vi "ProstateThumbnails.vi"(5 "Log scaling?":bool, 6 "single frame?":bool, 7 "Data":i16[][][](array[numeric]), 9 "Overlay Co-Ords":T2 {"y overlay" format="%.2f"; "x overlay" format="%.2f"}, 10 "output cluster":T1={"header info"={"Header"="", "Head length"=0}, "A/D info"={"# rf points per line"=0, "# lines per scan"=0, "sample rate MHz"=0, "# A/D bits"=0, "# bytes per A/D"=0, "TGC Flag"=0, "A/D Type"=""}, "Tranducer Info"={"bandwidth"=0.0, "center freq"=0.0, "start freq"=0.0, "ID"=0}, "Scan Info"={"delay"=0.0, "pivot distance"=0.0, "sector scan angle"=0.0, "operator"="", "Scan Mode"="", "location"=""}, "Time/Date Info"={"date"="", "time"=""}, "RF Info"={"RF file name"="", "RF file att"="", "RF cal file name"="", "RF cal file att"=""}, "Patient Info"={"ID"="", "extended ID"="", "age"=0, "sex"="", "previously\nscanned"="", "PSA"=0.0, "LOS"=1, "Ethnicty 2"=3, "Race"=3}, "Tissue Type"={"organ"=0, "disease type"=0, "disease location"=0, "IQ_pts"=0, "RcvBuffer"=0, "RcvFrame"=0, "IQBuff"=0, "IQFrame"=0, "IQPage"=0}, "Votage scaling"={"Digitizer (dB)"=0.0, "Gain (dB)"=0.0, "Atten (dB)"=0.0}, "Comment"="", "Misc Info"={"avg num"=0, "c speed"=0, "Div By or SF zones"=0, "XMIT CHS"=0, "RCV CHS"=0, "Xmit angle"=0.0}, "Therapy Parameters"={"Theraputic Freq (MHz)"=0.1, "Time on (s)"=1.0, "Therapy amplitude (mV)"=50.0, "Lines Before"=20, "Lines After"=80}, "Scan Settings"={"Energy (uJ or V)"=0, "Damp (Ohm) or Fc"=0, "HP Filt (KHz)"=0, "LP Filt (MHz)"=0, "Gain (db)"=0, "prf (kHz)"=0.0, "Distance between\nscan lines (um)"=0, "Distance between\nscan planes (um)"=0, "Scan line gap (um)"=0.0, "Scan plane gap (um)"=0.0}, "Compression Parameters"={"F1 (MHz)"=0.0, "F2 (MHz)"=0.0, "% taper"=0.0, "duration"=0.0}, "Patient Info Xtra"={"First Name"="", "Last Name"="", "Notes"=""}, "ROI Box"=[0, 0, 0, 0]} {"Compression Parameters"."% taper" min=50 max=1000 format="%.2f"; "Compression Parameters"."F2 (MHz)" format="%.3f"; "Compression Parameters"."F1 (MHz)" format="%.3f"; "Scan Settings"."prf (kHz)" format="%.2f"; "Therapy Parameters"."Therapy amplitude (mV)" min=50 max=1000 format="%.2f"; "Therapy Parameters"."Time on (s)" format="%.3f"; "Therapy Parameters"."Theraputic Freq (MHz)" format="%.3f"; "Patient Info"."Race" items=["Am Ind or Alaska", "Asian", "Hawaiian, Pac Isl", "Black or Afr Amer", "White", "more than one race", "unknown"]; "Patient Info"."Ethnicty 2" items=["Hispanic", "Non-Hispanic", "unknown"]; "Patient Info"."LOS" items=["1", "2", "3", "4", "5"]; "Patient Info"."PSA" format="%.1f"; "Scan Info"."delay" format="%.2f"; "Scan Info"."pivot distance" format="%.2f"; "Scan Info"."sector scan angle" format="%.2f"; "Tranducer Info"."bandwidth" format="%.2f"; "Tranducer Info"."center freq" format="%.2f"; "Tranducer Info"."start freq" format="%.2f"}, 11 "Thumb Size":cluster{"pixels in x":i16, "pixels in y":i16}) -> (3 "Thumbs out":picture[](array[picture]))   [LabVIEW 2022 SP3]
uses:
  ViewData/-ReadEye/Header.ctl
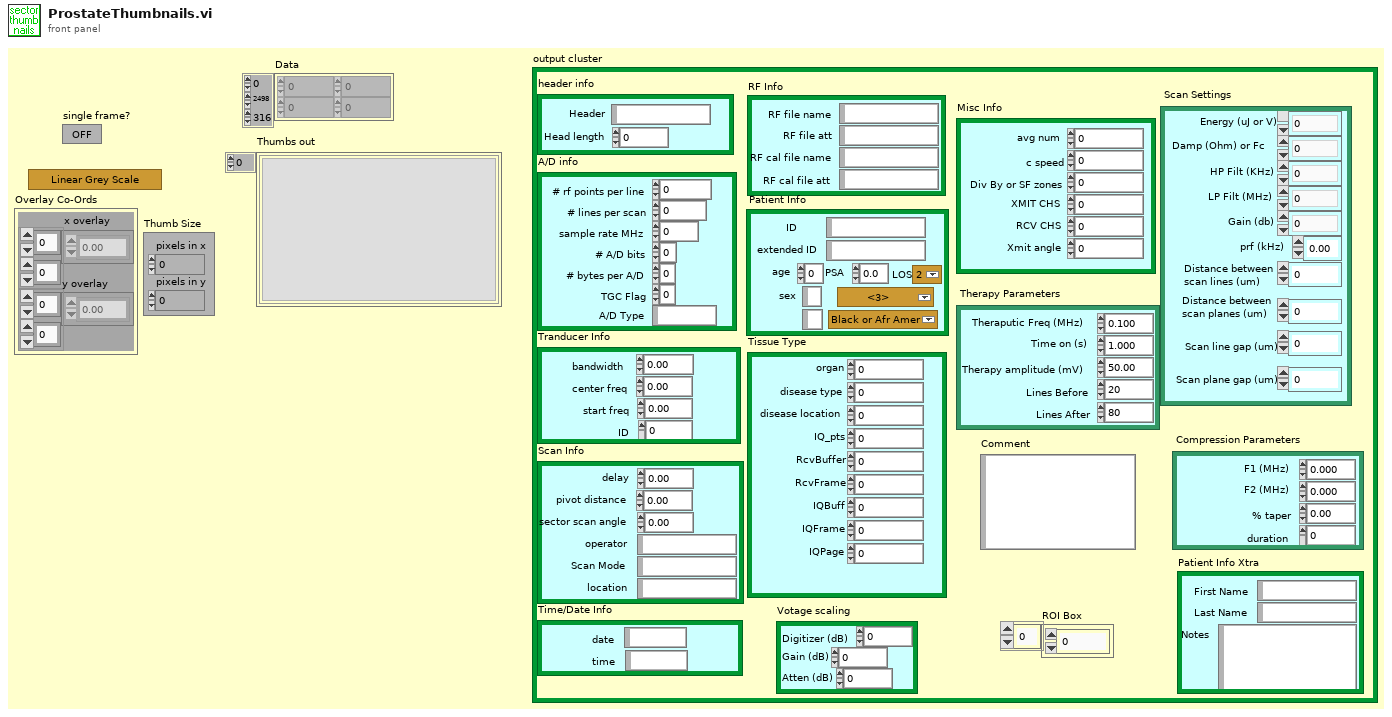
[diagram p1: front panel]
types:
  T1 = typedef "Header.ctl" = cluster{"header info":cluster{"Header":string, "Head length":i16}, "A/D info":cluster{"# rf points per line":u16, "# lines per scan":u16, "sample rate MHz":u16, "# A/D bits":i16, "# bytes per A/D":u16, "TGC Flag":u16, "A/D Type":string}, "Tranducer Info":cluster{"bandwidth":sgl, "center freq":sgl, "start freq":sgl, "ID":i32}, "Scan Info":cluster{"delay":sgl, "pivot distance":sgl, "sector scan angle":sgl, "operator":string, "Scan Mode":string, "location":string}, "Time/Date Info":cluster{"date":string, "time":string}, "RF Info":cluster{"RF file name":string, "RF file att":string, "RF cal file name":string, "RF cal file att":string}, "Patient Info":cluster{"ID":string, "extended ID":string, "age":u16, "sex":string, "previously\nscanned":string, "PSA":sgl, "LOS":u8, "Ethnicty 2":u8, "Race":u8}, "Tissue Type":cluster{"organ":i16, "disease type":i16, "disease location":i16, "IQ_pts":u16, "RcvBuffer":u8, "RcvFrame":u16, "IQBuff":u8, "IQFrame":u16, "IQPage":u8}, "Votage scaling":cluster{"Digitizer (dB)":sgl, "Gain (dB)":sgl, "Atten (dB)":sgl}, "Comment":string, "Misc Info":cluster{"avg num":u16, "c speed":i16, "Div By or SF zones":i16, "XMIT CHS":u8, "RCV CHS":u8, "Xmit angle":sgl}, "Therapy Parameters":cluster{"Theraputic Freq (MHz)":sgl, "Time on (s)":sgl, "Therapy amplitude (mV)":sgl, "Lines Before":u16, "Lines After":u16}, "Scan Settings":cluster{"Energy (uJ or V)":u8, "Damp (Ohm) or Fc":u8, "HP Filt (KHz)":u8, "LP Filt (MHz)":u8, "Gain (db)":u8, "prf (kHz)":sgl, "Distance between\nscan lines (um)":u16, "Distance between\nscan planes (um)":u16, "Scan line gap (um)":sgl, "Scan plane gap (um)":sgl}, "Compression Parameters":cluster{"F1 (MHz)":sgl, "F2 (MHz)":sgl, "% taper":sgl, "duration":sgl}, "Patient Info Xtra":cluster{"First Name":string, "Last Name":string, "Notes":string}, "ROI Box":u16[]}
  T2 = cluster{"x overlay":dbl[][], "y overlay":dbl[][]}
  T3 = cluster{"Font Name:":string, "Size":i16, "Strikeout?":bool, "Italic?":bool, "Underline?":bool, "Outline?":bool, "Shadow?":bool, "Bold?":bool}
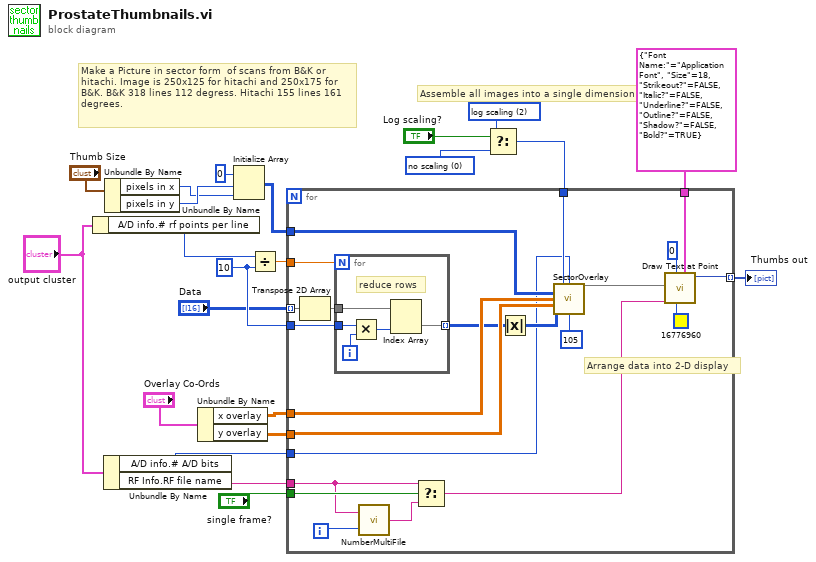
[diagram p0: block diagram]
diagram:
  w10 = u16 0 items=["no scaling", "scale to 255", "log scaling"] ("scaling")
  w11 = u16 2 items=["no scaling", "scale to 255", "log scaling"] ("scaling")
  w6 = 10
  # "Make a Picture in sector form  of scans from B&K or hitachi. Image is 250x125 for hitachi and 250x175 for B&K. B&K 318 lines 112 degress. Hitachi 155 lines 161 degrees."
  # "Assemble all images into a single dimension array."
  n1 = Unbundle By Name("output cluster") -> ("A/D info.# rf points per line"=w7:u16)
  n2 = Unbundle By Name("output cluster") -> ("A/D info.# A/D bits"=w9:i16, "RF Info.RF file name"=w21:string)
  n3 = Unbundle By Name("Thumb Size") -> ("pixels in x"=w12:i16, "pixels in y"=w13:i16)
  n4 = Unbundle By Name("Overlay Co-Ords") -> ("x overlay"=w2:dbl[][], "y overlay"=w3:dbl[][])
  n5 = Initialize Array(i16 0, w13, w12) -> (w15:i16[][])
  n6 = Divide(x=w7, y=w6) -> (x/y=w8:dbl)
  n7 = Select(t=w11, s="Log scaling?", f=w10) -> (s? t:f=w19:u16)
  n8 = for {
    tunnel: "Data" -> [w24] mode=indexing
    tunnel: [w43] -> w18 mode=indexing
    tunnel: w21 -> [w40]
    tunnel: "single frame?" -> [w42]
    tunnel: w19 -> [w29]
    tunnel: T3 {"Font Name:"="Application Font", "Size"=18, "Strikeout?"=FALSE, "Italic?"=FALSE, "Underline?"=FALSE, "Outline?"=FALSE, "Shadow?"=FALSE, "Bold?"=TRUE} ("[user-specified font]") -> [w38]
    tunnel: w3 -> [w31]
    tunnel: w2 -> [w32]
    tunnel: w15 -> [w33]
    tunnel: w8 -> [w36]
    tunnel: w6 -> [w35]
    tunnel: w9 -> [w25]
    i -> [w34]
    # "Arrange data into 2-D display"
    n9 = Transpose 2D Array(2D array=w24) -> (transposed array=w23:i16[][])
    n10 = for {
      N: w36 -> [_]
      tunnel: w23 -> [w49]
      tunnel: w35 -> [w47]
      tunnel: [w46] -> w28 mode=indexing
      i -> [w48]
      # "reduce rows"
      n11 = Multiply(x=w47, y=w48) -> (x*y=w45:i32)
      n12 = Index Array(array=w49, index (col)=w45) -> (element=w46:i16[])  [unwired: 1 in]
    }
    n13 = call "NumberMultiFile.vi"("File number"=w34, "file name"=w40) -> ("Numbered File"=w41:string)
    n14 = Select(t=w40, s=w42, f=w41) -> (s? t:f=w39:string)
    n15 = Absolute Value(x=w28) -> (abs(x)=w26:i16[][])
    n16 = call "SectorOverlay.vi"("Abs?"=w29, "Interp Mode"=w25, "Empty Array"=w33, "x Scaled"=w32, "y Scaled"=w31, "z values"=w26, 13:105) -> (4:w30)  [unwired: 2 in, 6 out]
    n17 = call <vilib>:"Draw Text at Point.vi"("[user-specified font]"=w38, "text color(black)"=u32 16776960, "desired font(Application)"=0, "text"=w39, "picture"=w30) -> ("new picture"=w43:picture)  [unwired: 4 in, 2 out]
  }
  "Thumbs out" <- w18
